vi "oax_Freq-RPM Map.vi"() -> ()   [LabVIEW 2017]
doc: "This VI is a sub-window of Order Analyzer. It displays RPM-Order map in intensity graph and waterfall plot."
uses:
  <vilib>/addons/Sound and Vibration/Order Analysis/Ref Gabor Order Tracking/Get Freq-RPM Spectral Map (DBL).vi
  <vilib>/addons/Sound and Vibration/Order Analysis/Ref Gabor Order Tracking/Get Freq-RPM Spectral Map (U8).vi
  <vilib>/addons/Sound and Vibration/Order Analysis/Example Support/Demo VI/Start-Up Kit/OAT Start/global variable.vi
  <vilib>/addons/Sound and Vibration/Order Analysis/Gabor Order Tracking/SoundVib_Gabor.lvlib
panel:
  out "size(s)":i32[](array[numeric])
  in  "Reference Level":dbl=40.0 caption="EU"
  in  "help mask":cluster{"OK Button":bool}
  in  "Help":bool
  out "Cursor Mask":cluster{dbl, dbl}[](graph)=[{0.0, 0.0}, {1027.7777297297296, 512.0}]
  out "Diagram":picture
  out "Freq-RPM Map":u8[][](graph)
  in  "[user-specified font]":T1={"Font Name:"="MS Sans Serif", "Size"=13, "Strikeout?"=FALSE, "Italic?"=FALSE, "Underline?"=FALSE, "Outline?"=FALSE, "Shadow?"=FALSE, "Bold?"=FALSE}
  out "Order":dbl=29.88973112705829 format="%.1f"
  in  "Order Info":T2={"Lowest order"=1.0, "# of Orders"=20.0, "Resolution"=0.1} {"Resolution" format="%.2f"; "# of Orders" format="%.1f"; "Lowest order" format="%.1f"}
  in  "dB ON":bool=TRUE
  in  "Waterfall ColorMap":i32(ring)=2 items=["cwNone", "cwShaded", "cwColorSpectrum", "cwGrayScale"]
  out "status":string
  in  "Diagram\n\nIntensity":bool
  # "1. Zoom Intensity Graph by setting ranges of axis.\n\n2. Switch to Diagram to display Campbell diagram.\n\n3. Move the cursor to find out which order the engergy consentrats on.\n\nClick on this screen to continue"
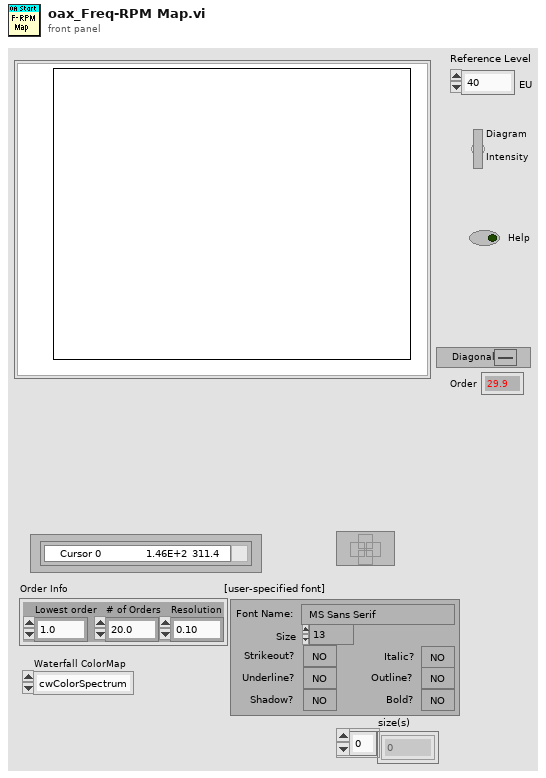
[diagram p1: front panel]
types:
  T1 = cluster{"Font Name:":string, "Size":i16, "Strikeout?":bool, "Italic?":bool, "Underline?":bool, "Outline?":bool, "Shadow?":bool, "Bold?":bool}
  T2 = cluster{"Lowest order":dbl, "# of Orders":dbl, "Resolution":dbl}
  T3 = enum16{"User-specified Font", "Application Font", "System Font", "Dialog Font"}
  T4 = cluster{"x minimum":dbl, "x maximum":dbl, "x log?":bool, "x precision":u8, "x format":enum8{"Decimal", "Scientific", "Engineering", "Binary", "Octal", "Hex"}, "y minimum":dbl, "y maximum":dbl, "y log?":bool, "y precision":u8, "y format":enum8{"Decimal", "Scientific", "Engineering", "Binary", "Octal", "Hex"}}
  T5 = typedef "SoundVib_Gabor.lvlib/GT RefNum.ctl" = refnum<k1>
  T6 = cluster{"Gabor RefNum":T5, "dB ON":bool, "Order Info":cluster{"Lowest order":dbl, "# of Orders":dbl, "Resolution":dbl}}
  T7 = cluster{"Diagram\n\nIntensity":bool, "Waterfall ColorMap":i32, "Reference Level":dbl}
  T8 = typedef "LVBoundsTypeDef.ctl" = cluster{"Width":u32, "Height":u32}
  T9 = cluster{"x [EU]":dbl, "y [EU]":dbl, "radius [pixel]":dbl}[]
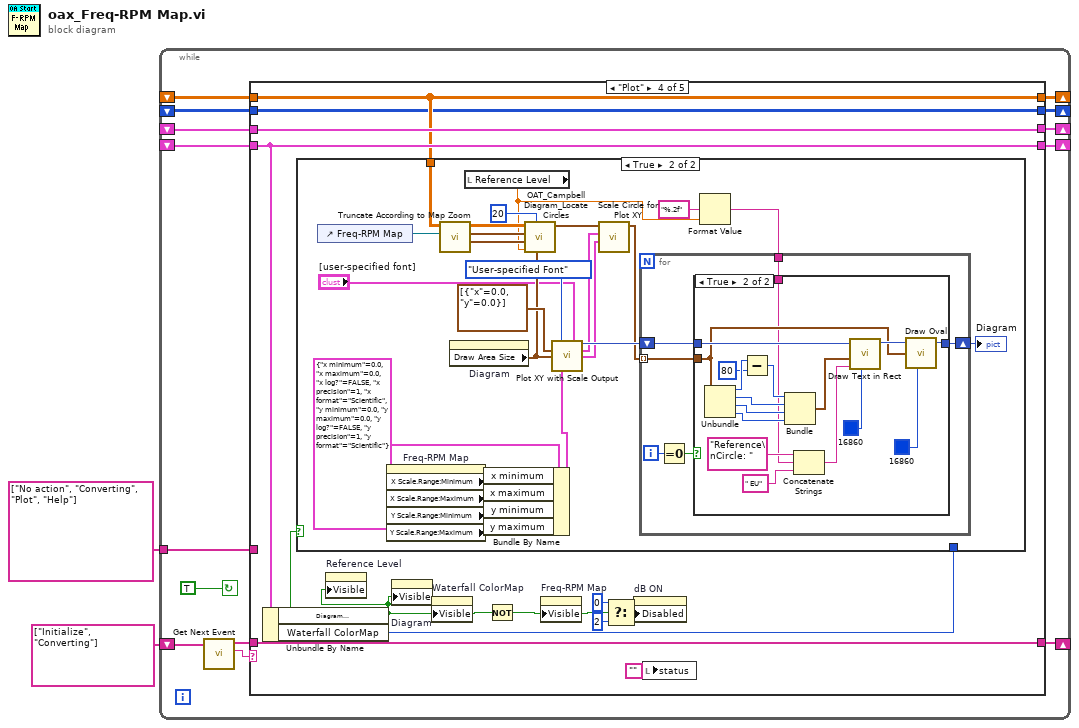
[diagram p0: block diagram]
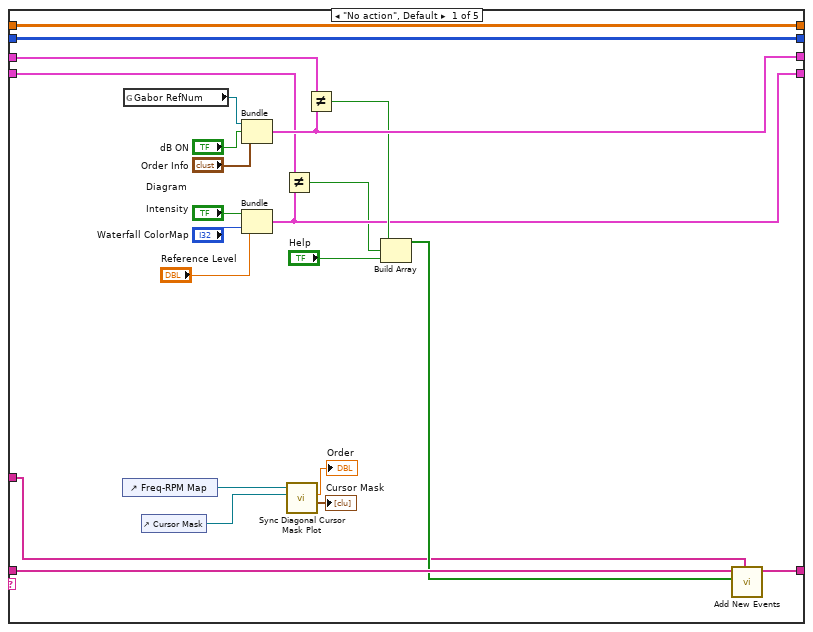
[diagram p2: hidden frame]
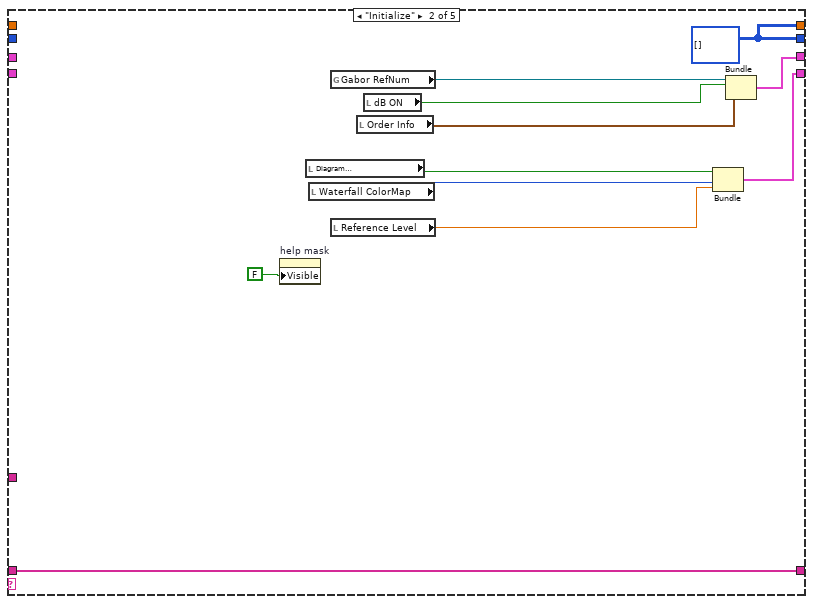
[diagram p3: hidden frame]
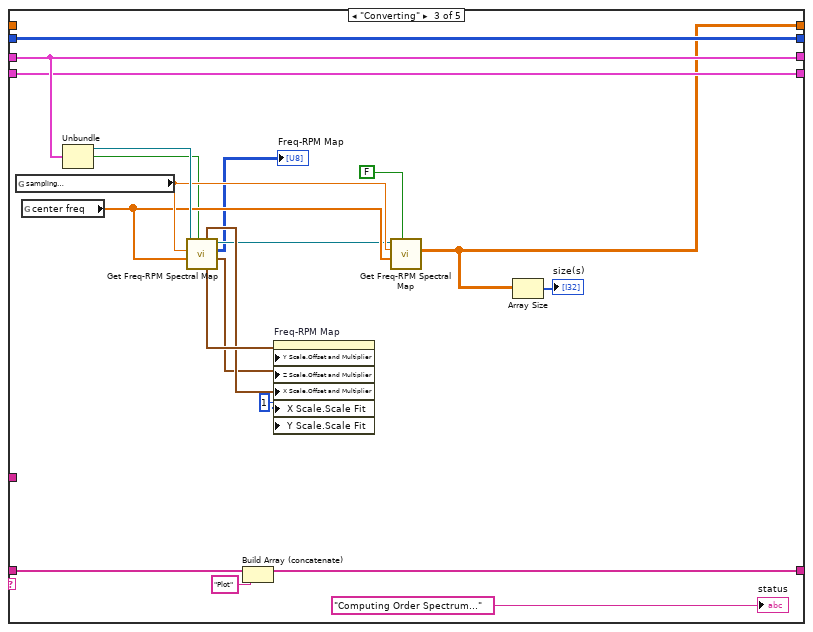
[diagram p4: hidden frame]
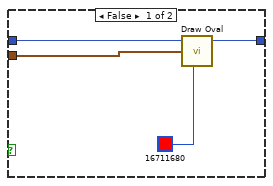
[diagram p6: hidden frame]
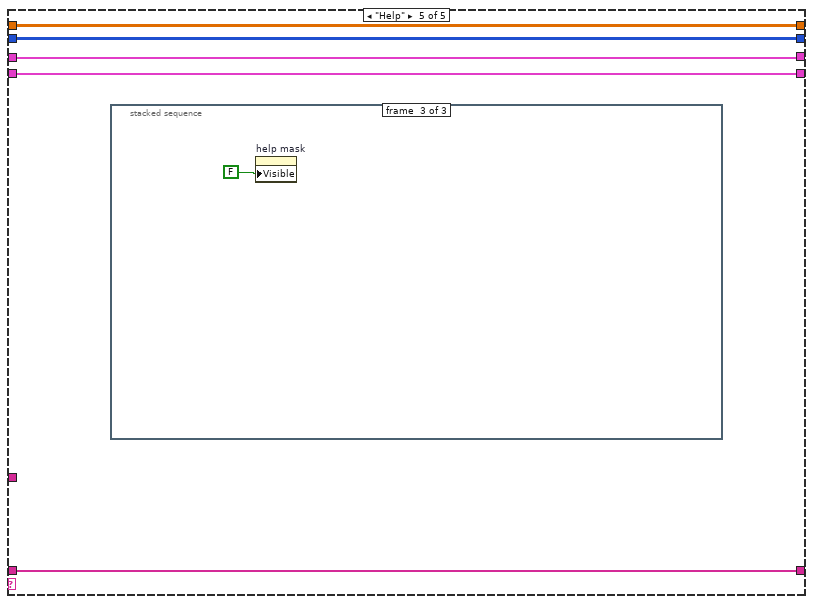
[diagram p7: hidden frame]
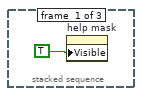
[diagram p8: hidden frame]
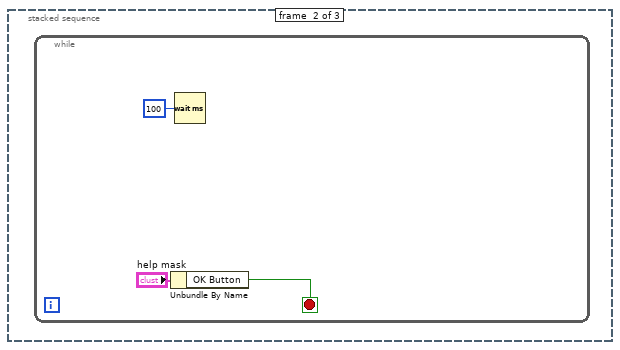
[diagram p9: hidden frame]
diagram:
  n1 = while {
    shift-left: _ -> [w3]
    shift-right: [w4] -> _
    tunnel: string[] ["No action", "Converting", "Plot", "Help"] ("Event Queue Out") -> [w5]
    shift-left: _ -> [w7]
    shift-right: [w6] -> _
    shift-left: _ -> [w8]
    shift-right: [w9] -> _
    shift-left: _ -> [w10]
    shift-right: [w11] -> _
    shift-left: string[] ["Initialize", "Converting"] ("Event Queue Out") -> [w12]
    shift-right: [w15] -> _
    stop <- TRUE continue-if-true
    n2 = call <vilib>:"Get Next Event.vi"("Event Queue In"=w12) -> ("Next Event"=w13:string, "Event Queue Out"=w14:string[])  [unwired: 5 in]
    n3 = case shown="\"Plot\"" w13 {
      tunnel: [w39 w42 w54 w72 w138] -> w11
      tunnel: w10 -> [w39 _ w54 w72 w138]
      tunnel: [w38 w50 w68 w81 w135] -> w15
      tunnel: w14 -> [w37 w50 w70 w81 w135]
      tunnel: [w34 w47 w67 w78 w137] -> w9
      tunnel: w8 -> [w33 _ w67 w78 w137]
      tunnel: w7 -> [w29 _ w65 w82 w136]
      tunnel: [w28 w44 w65 w82 w136] -> w6
      tunnel: w5 -> [w25 _ _ _ _]
      tunnel: [w19 w42 w52 w76 w139] -> w4
      tunnel: w3 -> [w19 _ _ w76 w139]
      frame "No action", Default {
        n4 = control-ref of="Freq-RPM Map"() -> (w23:refnum<vi>)
        n5 = global read "global variable.vi" "Gabor RefNum"() -> (w36:T5)
        n6 = control-ref of="Cursor Mask"() -> (w22:refnum<vi>)
        n7 = Bundle("Gabor RefNum"=w36, "dB ON"="dB ON", "Order Info"="Order Info") -> (w34:T6)  [unwired: 1 in]
        n8 = Bundle("Diagram\n\nIntensity"="Diagram\n\nIntensity", "Waterfall ColorMap"="Waterfall ColorMap", "Reference Level"="Reference Level") -> (w28:T7)  [unwired: 1 in]
        n9 = Not Equal?(x=w29, y=w28) -> (x != y?=w26:bool)
        n10 = call <vilib>:"Sync Diagonal Cursor Mask Plot.vi"("Cursor Mask"=w22, "Freq-RPM Map"=w23) -> ("diagonal line"=→"Cursor Mask":cluster{dbl, dbl}[], "order number"=→"Order":dbl)  [unwired: 7 in, 1 out]
        n11 = Not Equal?(x=w33, y=w34) -> (x != y?=w32:bool)
        n12 = Build Array(w32, w26, "Help") -> (w27:bool[])
        n13 = call <vilib>:"Add New Events.vi"("Event Names"=w25, "New Events"=w27, "Event Queue In"=w37) -> ("Event Queue Out"=w38:string[])  [unwired: 8 in]
      }
      frame "Initialize" {
        w42 = u8[][] [] ("Graph Data [U8]")
        n14 = property on="help mask" class="Clust"("Visible"=FALSE) -> ()  [unwired: 2 in, 2 out]
        n15 = local read "Diagram\n\nIntensity"() -> (w45:bool)
        n16 = local read "Waterfall ColorMap"() -> (w46:i32)
        n17 = global read "global variable.vi" "Gabor RefNum"() -> (w48:T5)
        n18 = local read "Reference Level"() -> (w40:dbl)
        n19 = local read "Order Info"() -> (w43:T2)
        n20 = local read "dB ON"() -> (w49:bool)
        n21 = Bundle("Diagram\n\nIntensity"=w45, "Waterfall ColorMap"=w46, "Reference Level"=w40) -> (w44:T7)  [unwired: 1 in]
        n22 = Bundle("Gabor RefNum"=w48, "dB ON"=w49, "Order Info"=w43) -> (w47:T6)  [unwired: 1 in]
      }
      frame "Converting" {
        w55 = u8 1 ("Z Scale.Scale Fit")
        n23 = global read "global variable.vi" "sampling \nfrequency (Hz)"() -> (w63:dbl)
        n24 = global read "global variable.vi" "center freq"() -> (w62:dbl[])
        n25 = Unbundle(w67) -> ("Gabor RefNum"=w64:T5, "dB ON"=w56:bool)  [unwired: 1 out]
        n26 = call-poly <vilib>:"Get Freq-RPM Spectral Map.vi"("dB On (T)"=w56, "Gabor template"=w62, "sampling frequency [Hz]"=w63, "RefNum in"=w64) -> ("quantization info"=w59:cluster{"offset":dbl, "multiplier":dbl}, "spectral map"=→"Freq-RPM Map":u8[][], "RefNum out"=w58:T5, "frequency scale"=w61:cluster{"offset":dbl, "multiplier":dbl}, "rpm scale"=w60:cluster{"offset":dbl, "multiplier":dbl})  [unwired: 2 in, 1 out]
        n27 = Build Array (concatenate)(w70, "Plot" ("status")) -> (w68:string[])
        n28 = property on="Freq-RPM Map" class="IntGraph (strict)"("Y Scale.Offset and Multiplier"=w61, "Z Scale.Offset and Multiplier"=w59, "X Scale.Offset and Multiplier"=w60, "X Scale.Scale Fit"=w55, "Y Scale.Scale Fit"=w55) -> ()  [unwired: 2 in, 2 out]
        n29 = call-poly <vilib>:"Get Freq-RPM Spectral Map.vi"("dB On (T)"=FALSE, "Gabor template"=w62, "sampling frequency [Hz]"=w63, "RefNum in"=w58) -> ("spectral map"=w52:dbl[][])  [unwired: 2 in, 5 out]
        n30 = Array Size(array=w52) -> (size(s)=→"size(s)":i32[])
        "status" <- "Computing Order Spectrum..."
      }
      frame "Plot" {
        n31 = Unbundle By Name(w82) -> ("Diagram\n\nIntensity"=w71:bool, "Waterfall ColorMap"=w79:i32)
        n32 = case shown="True" w71 {
          tunnel: w76 -> [_ w90]
          tunnel: w79 -> [_ _]
          frame False {
          }
          frame True {
            n33 = control-ref of="Freq-RPM Map"() -> (w83:refnum<vi>)
            n34 = property on="Freq-RPM Map" class="IntGraph (strict)"() -> ("X Scale.Range:Minimum"=w107:dbl, "X Scale.Range:Maximum"=w106:dbl, "Y Scale.Range:Minimum"=w105:dbl, "Y Scale.Range:Maximum"=w104:dbl)  [unwired: 2 in, 2 out]
            n35 = call <vilib>:"Truncate According to Map Zoom.vi"("Map reference"=w83, "data"=w90) -> ("Y Scale.Offset and Multiplier"=w87:cluster{"Offset":dbl, "Multiplier":dbl}, "X Scale.Offset and Multiplier"=w88:cluster{"Offset":dbl, "Multiplier":dbl}, "data out"=w89:dbl[][])  [unwired: 7 in]
            n36 = property on="Diagram" class="Pict"() -> ("Draw Area Size"=w96:T8)  [unwired: 2 in, 2 out]
            n37 = local read "Reference Level"() -> (w85:dbl)
            n38 = Bundle By Name(cluster=T4 {"x minimum"=0.0, "x maximum"=0.0, "x log?"=FALSE, "x precision"=1, "x format"=enum."Scientific", "y minimum"=0.0, "y maximum"=0.0, "y log?"=FALSE, "y precision"=1, "y format"=enum."Scientific"} ("cartesian axis attributes"), "x minimum"=w107, "x maximum"=w106, "y minimum"=w105, "y maximum"=w104) -> (w103:T4)
            n39 = call <vilib>:"OAT_Campbell Diagram_Locate Circles.vi"("picture size (w,h)"=w96, "number of x steps"=20, "Reference Level"=w85, "y scale"=w87, "x scale"=w88, "map"=w89) -> ("circles"=w95:T9)  [unwired: 5 in]
            n40 = call <vilib>:"Plot XY with Scale Output.vi"("desired font(Application)"=T3."User-specified Font", "[user-specified font]"="[user-specified font]", "data"=cluster{"x":dbl, "y":dbl}[] [{"x"=0.0, "y"=0.0}], "dimensions (w,h)"=w96, "cartesian axis attributes"=w103) -> ("new picture"=w101:picture, "x scale factors"=w99:cluster{"a":dbl, "b":dbl, "log?":bool}, "y scale factors"=w98:cluster{"a":dbl, "b":dbl, "log?":bool})  [unwired: 8 in]
            n41 = call <vilib>:"Scale Circle for Plot XY.vi"("y scale factors"=w98, "x scale factors"=w99, "circles"=w95) -> ("rectangles"=w97:cluster{i16, i16, i16, i16}[])  [unwired: 8 in]
            n42 = Format Value(format string="%.2f", value (0)=w85) -> (output string=w86:string)  [unwired: 1 in]
            n43 = for {
              shift-right: [w109] -> w100
              shift-left: w101 -> [w111]
              tunnel: w97 -> [w110] mode=indexing
              tunnel: w86 -> [w108]
              i -> [w113]
              n44 = Equal To 0?(x=w113) -> (x = 0?=w112:bool)
              n45 = case shown="True" w112 {
                tunnel: w111 -> [w117 w134]
                tunnel: w110 -> [w116 w126]
                tunnel: [w115 w131] -> w109
                tunnel: w108 -> [_ w119]
                frame False {
                  n46 = call <vilib>:"Draw Oval.vi"("picture"=w117, "rect"=w116, "color(black)"=u32 16711680) -> ("new picture"=w115:picture)  [unwired: 6 in]
                }
                frame True {
                  n47 = Unbundle(w126) -> (w129:i16, w122:i16, w124:i16, w125:i16)
                  n48 = Subtract(x=w129, y=i16 80) -> (x-y=w127:i16)
                  n49 = Bundle(w127, w122, w124, w125) -> (w123:cluster{i16, i16, i16, i16})  [unwired: 1 in]
                  n50 = Concatenate Strings("Reference\nCircle: " ("text"), w119, " EU" ("text")) -> (w120:string)
                  n51 = call <vilib>:"Draw Text in Rect.vi"("text color(black)"=u32 16860, "text"=w120, "rect"=w123, "picture"=w134) -> ("new picture"=w132:picture)  [unwired: 7 in]
                  n52 = call <vilib>:"Draw Oval.vi"("picture"=w132, "rect"=w126, "color(black)"=u32 16860) -> ("new picture"=w131:picture)  [unwired: 6 in]
                }
              }
            }
            "Diagram" <- w100
          }
        }
        n53 = property on="Reference Level" class="DigNum (strict)"("Visible"=w71) -> ()  [unwired: 2 in, 2 out]
        n54 = property on="Diagram" class="Pict"("Visible"=w71) -> ()  [unwired: 2 in, 2 out]
        n55 = property on="Waterfall ColorMap" class="Ring (strict)"("Visible"=w71) -> ()  [unwired: 2 in, 2 out]
        n56 = Not(x=w71) -> (.not. x?=w77:bool)
        n57 = property on="Freq-RPM Map" class="IntGraph (strict)"("Visible"=w77) -> ()  [unwired: 2 in, 2 out]
        n58 = Select(t=0, s=w77, f=2) -> (s? t:f=w75:i32)
        n59 = property on="dB ON" class="Bool (strict)"("Disabled"=w75) -> ()  [unwired: 2 in, 2 out]
        n60 = local write "status"("") -> ()
      }
      frame "Help" {
        n61 = stacked-sequence {
          frame #0 {
            n62 = property on="help mask" class="Clust"("Visible"=TRUE) -> ()  [unwired: 2 in, 2 out]
          }
          frame #1 {
            n63 = while {
              stop <- w142 stop-if-true
              n64 = Unbundle By Name("help mask") -> ("OK Button"=w142:bool)
              n65 = Wait (ms)(milliseconds to wait=u32 100) -> ()  [unwired: 1 out]
            }
          }
          frame #2 {
            n66 = property on="help mask" class="Clust"("Visible"=FALSE) -> ()  [unwired: 2 in, 2 out]
          }
        }
      }
    }
  }
